vi "Sine_Trajectory_simple.vi"(1 "Frequencies":dbl[](array[numeric]), 2 "Duration (s)":dbl, 3 "Period (s)":dbl, 4 "Amplitude":dbl) -> (0 "Combined Sine Pattern":dbl[](array[numeric]))   [LabVIEW 2015]
uses:
  <vilib>/Analysis/NI_AALBase.lvlib
panel:
  # "Here needs to be 0.001 or so"
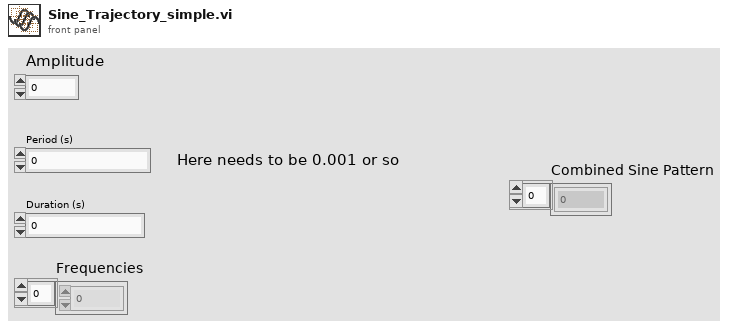
[diagram p1: front panel]
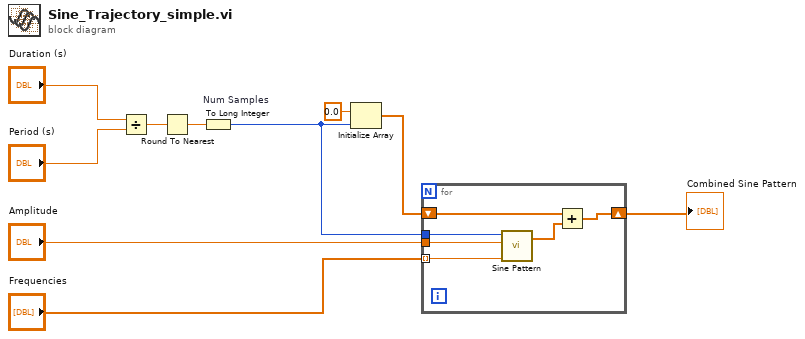
[diagram p0: block diagram]
diagram:
  n1 = Divide(x="Duration (s)", y="Period (s)") -> (x/y=w8:dbl)
  n2 = Round To Nearest(number=w8) -> (nearest integer value=w7:dbl)
  n3 = To Long Integer "Num Samples"(number=w7) -> (32bit integer=w4:i32)
  n4 = Initialize Array "Initialize Array"(0.0 ("element"), w4) -> (w2:dbl[])
  n5 = for {
    tunnel: "Frequencies" -> [w16] mode=indexing
    tunnel: w4 -> [w15]
    tunnel: "Amplitude" -> [w14]
    shift-right: [w13] -> w1
    shift-left: w2 -> [w11]
    n6 = call <vilib>:"Sine Pattern.vi"("cycles"=w16, "amplitude"=w14, "samples"=w15) -> ("Sinusoidal Pattern"=w12:dbl[])  [unwired: 1 in, 1 out]
    n7 = Add(x=w11, y=w12) -> (x+y=w13:dbl[])
  }
  "Combined Sine Pattern" <- w1
